vi "Fetch Digital Waveform Both.vi"(8 "error in (no error)":errorcluster {"code" format="%.0x"}, 11 "VISA Resource Name":refnum<visa-resource-name>) -> (0 "error out":errorcluster {"code" format="%.0x"}, 1 "x increment":dbl caption="x Increment" format="%^.2e", 2 "initial x":dbl caption="Initial x" format="%^.2e", 3 "VISA Resource Name Out":refnum<visa-resource-name>, 4 "waveform array":u16[](array[numeric]) caption="Waveform Array", 5 "actual points":u32 caption="Actual Points")   [LabVIEW 2011, in "Agilent 546XX Series.lvlib"]
doc: "This VI returns the waveform the oscilloscope acquires for the digital channel you specify. The waveform is from an acquisition that you previously initiated. \n\nYou use the ag546xx Initiate Acquisition VI to start an acquisition on the digital channels that you enable with the ag546xx Configure Digital Channel VI. The oscilloscope acquires waveforms for the enabled digital channels concurrently. You must call this VI separately for each enabled channel to obtain the waveforms.\n\nYou can call the ag546xx Read Digital Waveform VI instead of the ag546xx Initiate Acquisition VI. The ag546xx Read Digital Waveform VI starts an acquisition on all enabled channels, waits for the acquisition to complete, and returns the waveform for the channel you specify. You call this VI to obtain the value for all the digital channels in one waveform.\n\nNotes:\n\n(1) This VI returns the waveform of digital channels 0 to 15.\n\n(2) The Waveform Array is returned as an unsigned 16 bit number with digital channel 15 as the most significant bit and digital channel 0 as the least significant bit.\n\n(3) This VI is only used by models 546xx\"D\" models."
uses:
  Agilent 546XX Series.lvlib
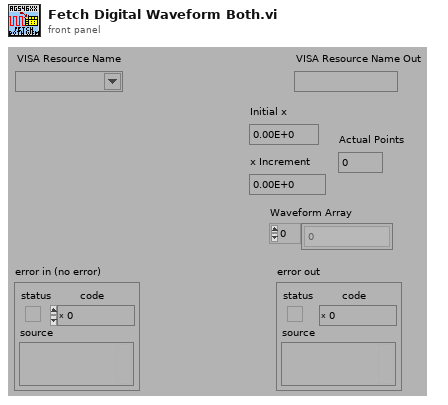
[diagram p1: front panel]
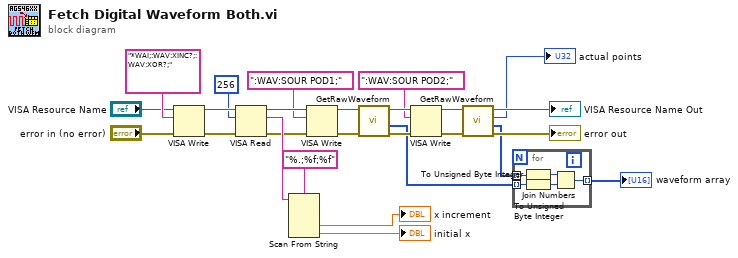
[diagram p0: block diagram]
diagram:
  n1 = VISA Write(VISA resource name="VISA Resource Name", write buffer="*WAI;:WAV:XINC?;:WAV:XOR?;", error in (no error)="error in (no error)") -> (VISA resource name out=w26:refnum<visa-resource-name>, error out=w25:errorcluster)  [unwired: 1 out]
  n2 = VISA Read(VISA resource name=w26, byte count=u32 256, error in (no error)=w25) -> (VISA resource name out=w18:refnum<visa-resource-name>, read buffer=w22:string, error out=w17:errorcluster)  [unwired: 1 out]
  n3 = Scan From String(format string="%.;%f;%f", input string=w22) -> (output 1=→"x increment":dbl, output 2=→"initial x":dbl)  [unwired: 4 in, 3 out]
  n4 = VISA Write(VISA resource name=w18, write buffer=":WAV:SOUR POD1;", error in (no error)=w17) -> (VISA resource name out=w16:refnum<visa-resource-name>, error out=w15:errorcluster)  [unwired: 1 out]
  n5 = call "GetRawWaveform.vi"("error in"=w15, "VISA Resource Name"=w16) -> ("error out"=w13:errorcluster, "Waveform Array"=w4:u32[], "VISA Resource Name Out"=w14:refnum<visa-resource-name>)  [unwired: 5 in, 2 out]
  n6 = VISA Write(VISA resource name=w14, write buffer=":WAV:SOUR POD2;", error in (no error)=w13) -> (VISA resource name out=w12:refnum<visa-resource-name>, error out=w11:errorcluster)  [unwired: 1 out]
  n7 = call "GetRawWaveform.vi"("error in"=w11, "VISA Resource Name"=w12) -> ("error out"=→"error out":errorcluster, "Waveform Array"=w5:u32[], "Number of Points"=→"actual points":u32, "VISA Resource Name Out"=→"VISA Resource Name Out":refnum<visa-resource-name>)  [unwired: 5 in, 1 out]
  n8 = for {
    tunnel: w5 -> [w27] mode=indexing
    tunnel: w4 -> [w29] mode=indexing
    tunnel: [w31] -> w3 mode=indexing
    n9 = To Unsigned Byte Integer(number=w27) -> (unsigned 8bit integer=w30:u8)
    n10 = To Unsigned Byte Integer(number=w29) -> (unsigned 8bit integer=w28:u8)
    n11 = Join Numbers(hi=w30, lo=w28) -> ((hi.lo)=w31:u16)
  }
  "waveform array" <- w3
